vi "Dashboard Main.vi"() -> ()   [LabVIEW 2018]
uses:
  Subsystems/Drive/MotionProfile/StartingPosition.ctl
  Subsystems/Drive/MotionProfile/Path_Decider.ctl
  <vilib>/Utility/miscctls.llb/LVRowAndColumnTypeDef.ctl
  <vilib>/event_ctls.llb/eventvkey.ctl
  <vilib>/Rock Robotics/Network Tables/NT Read Numeric Array.vi
  <vilib>/Rock Robotics/Network Tables/NT Read Boolean.vi
  <vilib>/Rock Robotics/Network Tables/NT Write Variant.vi
  <vilib>/Rock Robotics/WPI/Dashboard/WPI_DashboardLogging Global.vi
panel:
  out "lineIRRearRight":bool
  out "lineIRRearLeft":bool
  out "lineIRFrontRight":bool
  out "lineIRFrontLeft":bool
  out "climbSkidIRRight":bool
  out "climbSkidIRLeft":bool
  out "climbPoweredIRLeft":bool
  out "climbPoweredIRRight":bool
  in  "Camera Settings Right":T1={"Frame Rate"=30, "Compression"=30, "Size"=1, "DB Camera Config"=FALSE} {"Frame Rate" scale=1.0..30.0; "Compression" scale=100.0..-1.0; "Size" items=["640x480", "320x240", "160x120"]}
  in  "Camera Name Right":string(combo)="No Camera Selection"
  out "Camera Perf":string
  in  "Camera Settings":T1={"Frame Rate"=30, "Compression"=30, "Size"=1, "DB Camera Config"=FALSE} {"Frame Rate" scale=1.0..30.0; "Compression" scale=100.0..-1.0; "Size" items=["640x480", "320x240", "160x120"]}
  in  "TCP":refnum<k5>
  in  "Rec Mode":enum32{"Stop", "Record", "Playback"}(radio)
  out "Robot IP":string
  out "Image Message":string="Timeout in Camera Communications"
  in  "Dashboard Tab":T2(tab)
  in  "Select Auto":string(combo)="Select Autonomous ..."
  out "NT Connection":bool
  out "MotorChart R":cluster{"Numeric":dbl, "Numeric":dbl}(graph)
  out "MotorChart L":cluster{"Numeric":dbl, "Numeric":dbl}(graph)
  out "MotorSliders R":cluster{"MotorSlide1":dbl, "MotorSlide2":dbl} {"MotorSlide2" scale=-1.0..1.0 scale format="%#_2e"; "MotorSlide1" scale=-1.0..1.0 scale format="%#_2e"}
  out "MotorSliders L":cluster{"MotorSlide1":dbl, "MotorSlide2":dbl} {"MotorSlide2" scale=-1.0..1.0 scale format="%#_2e"; "MotorSlide1" scale=-1.0..1.0 scale format="%#_2e"}
  out "Gyro":dbl(knob) scale=0.0..360.0
  out "JS1 Z":dbl(slide) scale=-1.0..1.0 scale format="%#_2e"
  out "JS1 Graph":cluster{"X":dbl, "Y":dbl}[](graph)
  out "JS1 Buttons":T3
  out "JS2 Z":dbl(slide) scale=-1.0..1.0 scale format="%#_2e"
  out "JS2 Graph":cluster{"X":dbl, "Y":dbl}[](graph)
  out "JS2 Buttons":T3
  out "Mode":T4(ring)=enum."Auto Disabled"
  out "Right Camera Perf":cluster{"Bandwidth (Mbps)":dbl, "FPS":dbl}
  out "Camera Image Right":T5(plugin-control)
  in  "DB/String 9":string
  in  "DB/String 8":string
  in  "DB/String 7":string
  in  "DB/String 6":string
  in  "DB/String 5":string
  in  "DB/String 4":string
  in  "DB/String 3":string
  in  "DB/String 2":string
  in  "DB/String 1":string
  in  "DB/String 0":string
  in  "DB/Slider 0":dbl(slide) scale=0.0..5.0
  in  "DB/Slider 1":dbl(slide) scale=0.0..5.0
  in  "DB/Slider 2":dbl(slide) scale=0.0..5.0
  in  "DB/Slider 3":dbl(slide) scale=0.0..5.0
  out "DB/LED 3":bool
  out "DB/LED 2":bool
  out "DB/LED 1":bool
  out "DB/LED 0":bool
  in  "DB/Button 3":bool
  in  "DB/Button 2":bool
  in  "DB/Button 1":bool
  in  "DB/Button 0":bool caption="New Name"
  in  "Auto Options":T8={"Starting Position"=enum."Left L1 ", "First Score Pos"=enum."7", "Second Score Pos"=enum."5"}
  out "Waveform Chart":dbl(graph)
  out "HatchPanelDetect":bool
  in  "Test Slider":dbl(slide) scale=0.0..100.0 scale format="%#_3g"
  in  "On/Off":bool caption="Solenoid"
  in  "Test Name":u16(ring) items=["Select the test to run..."]
  in  "Test Tree":string(tree)
  in  "Motor":cluster{"Value":dbl, "Enable":bool} {"Value" scale=-1.0..1.0 scale format="%#_3g"}
  out "Progress":T9 {"Test Progress" scale=0.0..100.0}
  in  "Rev/Fwd":cluster{"Forward":bool, "Reverse":bool}
  in  "Test Ring":u16(ring) items=["Monochrome", "Color"]
  out "Cmd Status":string
  in  "Execute Command":bool
  in  "Command Params":string[][](table)
  in  "Command Selection":i32(listbox)
  in  "CheckList":i32(listbox)
  out "Tree":string(tree)
  out "Camera Image":T5(plugin-control)
  out "Background":bool
  in  "Camera Name":string(combo)="No Camera Selection"
  # "HW"
  # "HW"
  # "Joysticks"
  # "Drive Motors"
  # "Front"
  # "Right"
  # "Left"
  # "Back"
  # "This tab is a great place for autonomous settings and robot-specific values.\nPlace controls and indicators inside this tab and match name to\nDashboard Variables on robot. You can also delete this comment."
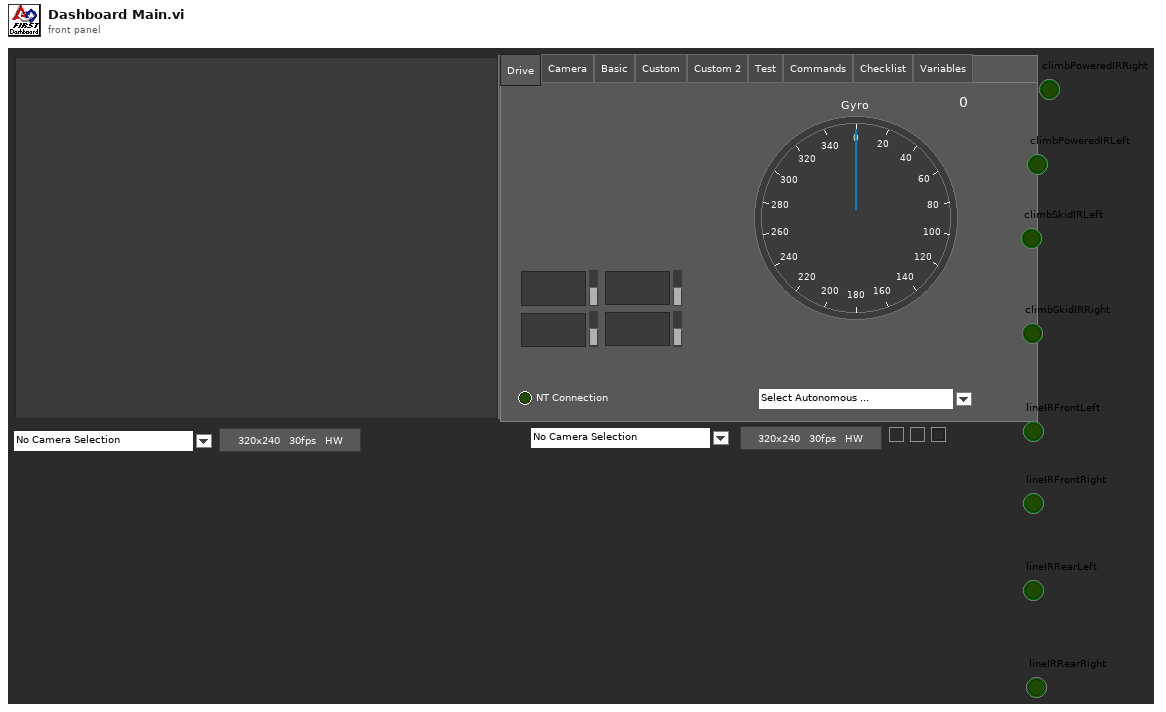
[diagram p1: front panel]
types:
  T1 = cluster{"Frame Rate":i32, "Compression":i32, "Size":u16, "DB Camera Config":bool}
  T2 = enum32{"Drive", "Camera", "Basic", "Custom", "Custom 2", "Test", "Commands", "Checklist", "Variables"}
  T3 = cluster{bool, bool, bool, bool, bool, bool, bool, bool, bool, bool, bool, bool}
  T4 = enum8{"Tele-Op Disabled", "Tele-Op Enabled", "Auto Disabled", "Auto Enabled", "Test Disabled", "Test Enabled", "Disconnected", "No Code", "E-Stop"}
  T5 = typedef "IMAQ Image.ctl" = refnum<image>
  T6 = typedef "StartingPosition.ctl" = enum16{"Left L1 ", "Middle L1", "Right L1", "Left L2", "Right L2", "Don't Move"}
  T7 = typedef "Path_Decider.ctl" = enum16{"1", "2", "3", "4", "5", "6", "7", "8", "Left_Rocket_Front", "Left_Rocket_Rear", "Right_Rocket_Front", "Right_Rocket_Rear"}
  T8 = cluster{"Starting Position":T6, "First Score Pos":T7, "Second Score Pos":T7}
  T9 = cluster{"Test Progress":u8, "Test Progress Text":string}
  T10 = cluster{"Save Path":path, "Interval (s)":dbl, "Keep":i32}
  T11 = enum32{"Drive", "Camera", "Basic", "Custom", "Test", "Commands", "Checklist", "Variables"}
  T12 = typedef "Image Type" = u32
  T13 = cluster{"IDs":cluster{"RPC field ID":u16, "Unique ID":u16}, "String":string}
  T14 = cluster{"Error Strings":string, "Disable Counts":cluster{u16, u16}, "Rail Faults":cluster{u16, u16, u16}, "Robot IP":string, "DB Mode":u8, "Event Info":cluster{"Name":string, "Type":u8, "Number":u16, "Replay":u8}}
  T15 = cluster{"Storage":cluster{"Disk Free":u64, "RAM Block":u32, "RAM free":u32}, "CPU Utilization":cluster{"CPU % ISR":sgl, "CPU % Time Crit":sgl, "CPU % Timed Str":sgl, "CPU % High":sgl, "CPU % Above":sgl, "CPU % Normal":sgl, "CPU % Low":sgl}, "CAN":cluster{"% Bus Utilization":sgl, "Bus Off Cnt":u32, "TX_FIFO Full Cnt":u32, "Receive Error Cnt":u8, "Transmit Error Cnt":u8}, "HID":cluster{"HID Outputs":u32, "Rumble Low":u16, "Rumble High":u16}[]}
  T16 = cluster{"Status bits":cluster{"Test Mode":bool, "Autonomous":bool, "Enabled":bool, "Code Start":bool, "Brownout":bool, "Reserved 2":bool, "Reserved 3":bool, "E-Stop":bool}, "Code Trace":cluster{"Disabled":bool, "TeleOp":bool, "Auto":bool, "Test":bool}, "Controller Type":enum16{"unknown", "cRIO", "roboRio"}, "Code?":enum16{"unknown", "noCode", "code"}, "Battery V":dbl}
  T17 = cluster{"Control Bits":cluster{"TestMode":bool, "Autonomous":bool, "Enabled":bool, "FMS Present":bool, bool, bool, bool, "E-Stop":bool}, "Team Station ":u8, "Countdown":sgl, "Joystick Values":cluster{"Axes":dbl[], "Buttons":bool[], "POVs":i16[]}[]}
  T18 = cluster{"Axes":dbl[], "Buttons":bool[], "POVs":i16[]}[]
  T19 = cluster{"Axes":dbl[], "Buttons":bool[], "POVs":i16[]}
  T20 = cluster{"Buttons[0]":bool, "Buttons[1]":bool, "Buttons[2]":bool, "Buttons[3]":bool, "Buttons[4]":bool, "Buttons[5]":bool, "Buttons[6]":bool, "Buttons[7]":bool, "Buttons[8]":bool, "Buttons[9]":bool, "Buttons[10]":bool, "Buttons[11]":bool}
  T21 = cluster{"Camera Image":refnum<vi>, "Dashboard Tab":refnum<vi>, "Background":refnum<vi>, "Rec Mode":refnum<vi>, "Test Slider":refnum<vi>, "On/Off ":refnum<vi>, "Test Ring":refnum<vi>, "Rev/Fwd":refnum<vi>, "Test Name":refnum<vi>, "Motor":refnum<vi>, "Progress":refnum<vi>, "CheckList":refnum<vi>, "Tree":refnum<vi>, "Test Tree":refnum<vi>, "Command Params":refnum<vi>, "Command Selection":refnum<vi>, "Execute Command":refnum<vi>, "Cmd Status":refnum<vi>, "Camera Settings":refnum<vi>, "Camera Name":refnum<vi>, "Camera Perf":refnum<vi>, "Camera Settings Right":refnum<vi>, "Camera Name Right":refnum<vi>, "Camera Image Right":refnum<vi>}
  T22 = cluster{"Global Rectangle":i32[], "Contours":cluster{"Contour Type":u32, "ROI Type":u32, "Points":i32[]}[]}
  T23 = cluster{"Camera Name Right":string, string, "Saved DB Images Info":cluster{"Save Path":path, "Interval (s)":dbl, "Keep":i32}}
  T24 = cluster{"Camera Name":string, string, "Saved DB Images Info":cluster{"Save Path":path, "Interval (s)":dbl, "Keep":i32}}
  T25 = cluster{"Operation":enum16{"Update", "Clear"}, "Color Box":u32}[]
  T26 = typedef "eventvkey.ctl" = enum16{"ASCII", "Enter", "Return", "Shift", "Ctrl", "Alt", "Cmd", "Opt", "Caps", "NumLock", "Clear", "Break", "Up", "Down", "Left", "Right", "Insert", "Delete", "Home", "End", "PageUp", "PageDown", "Escape", "Help", "Pause", "ScrollLock", "F1", "F2", "F3", "F4", "F5", "F6", "F7", "F8", "F9", "F10", "F11", "F12", "F13", "F14", "F15", "F16", "F17", "F18", "F19", "F20", "F21", "F22", "F23", "F24", "Play", "VolumeUp", "VolumeDown", "Mute", "Two Byte Char"}
  T27 = cluster{"Image Size":bool, "Image Type":bool, "Pixel Value":bool, "ROI Information":bool, "Zoom Factor":bool}
  T28 = cluster{"Operation":enum16{"Update", "Clear"}, "Color Box":u32}
  T29 = typedef "LVRowAndColumnTypeDef.ctl" = cluster{"Row":i32, "Column":i32}
  T30 = cluster{"Shift":bool, "Ctrl":bool, "Alt":bool, "Cmd":bool, "Opt":bool}
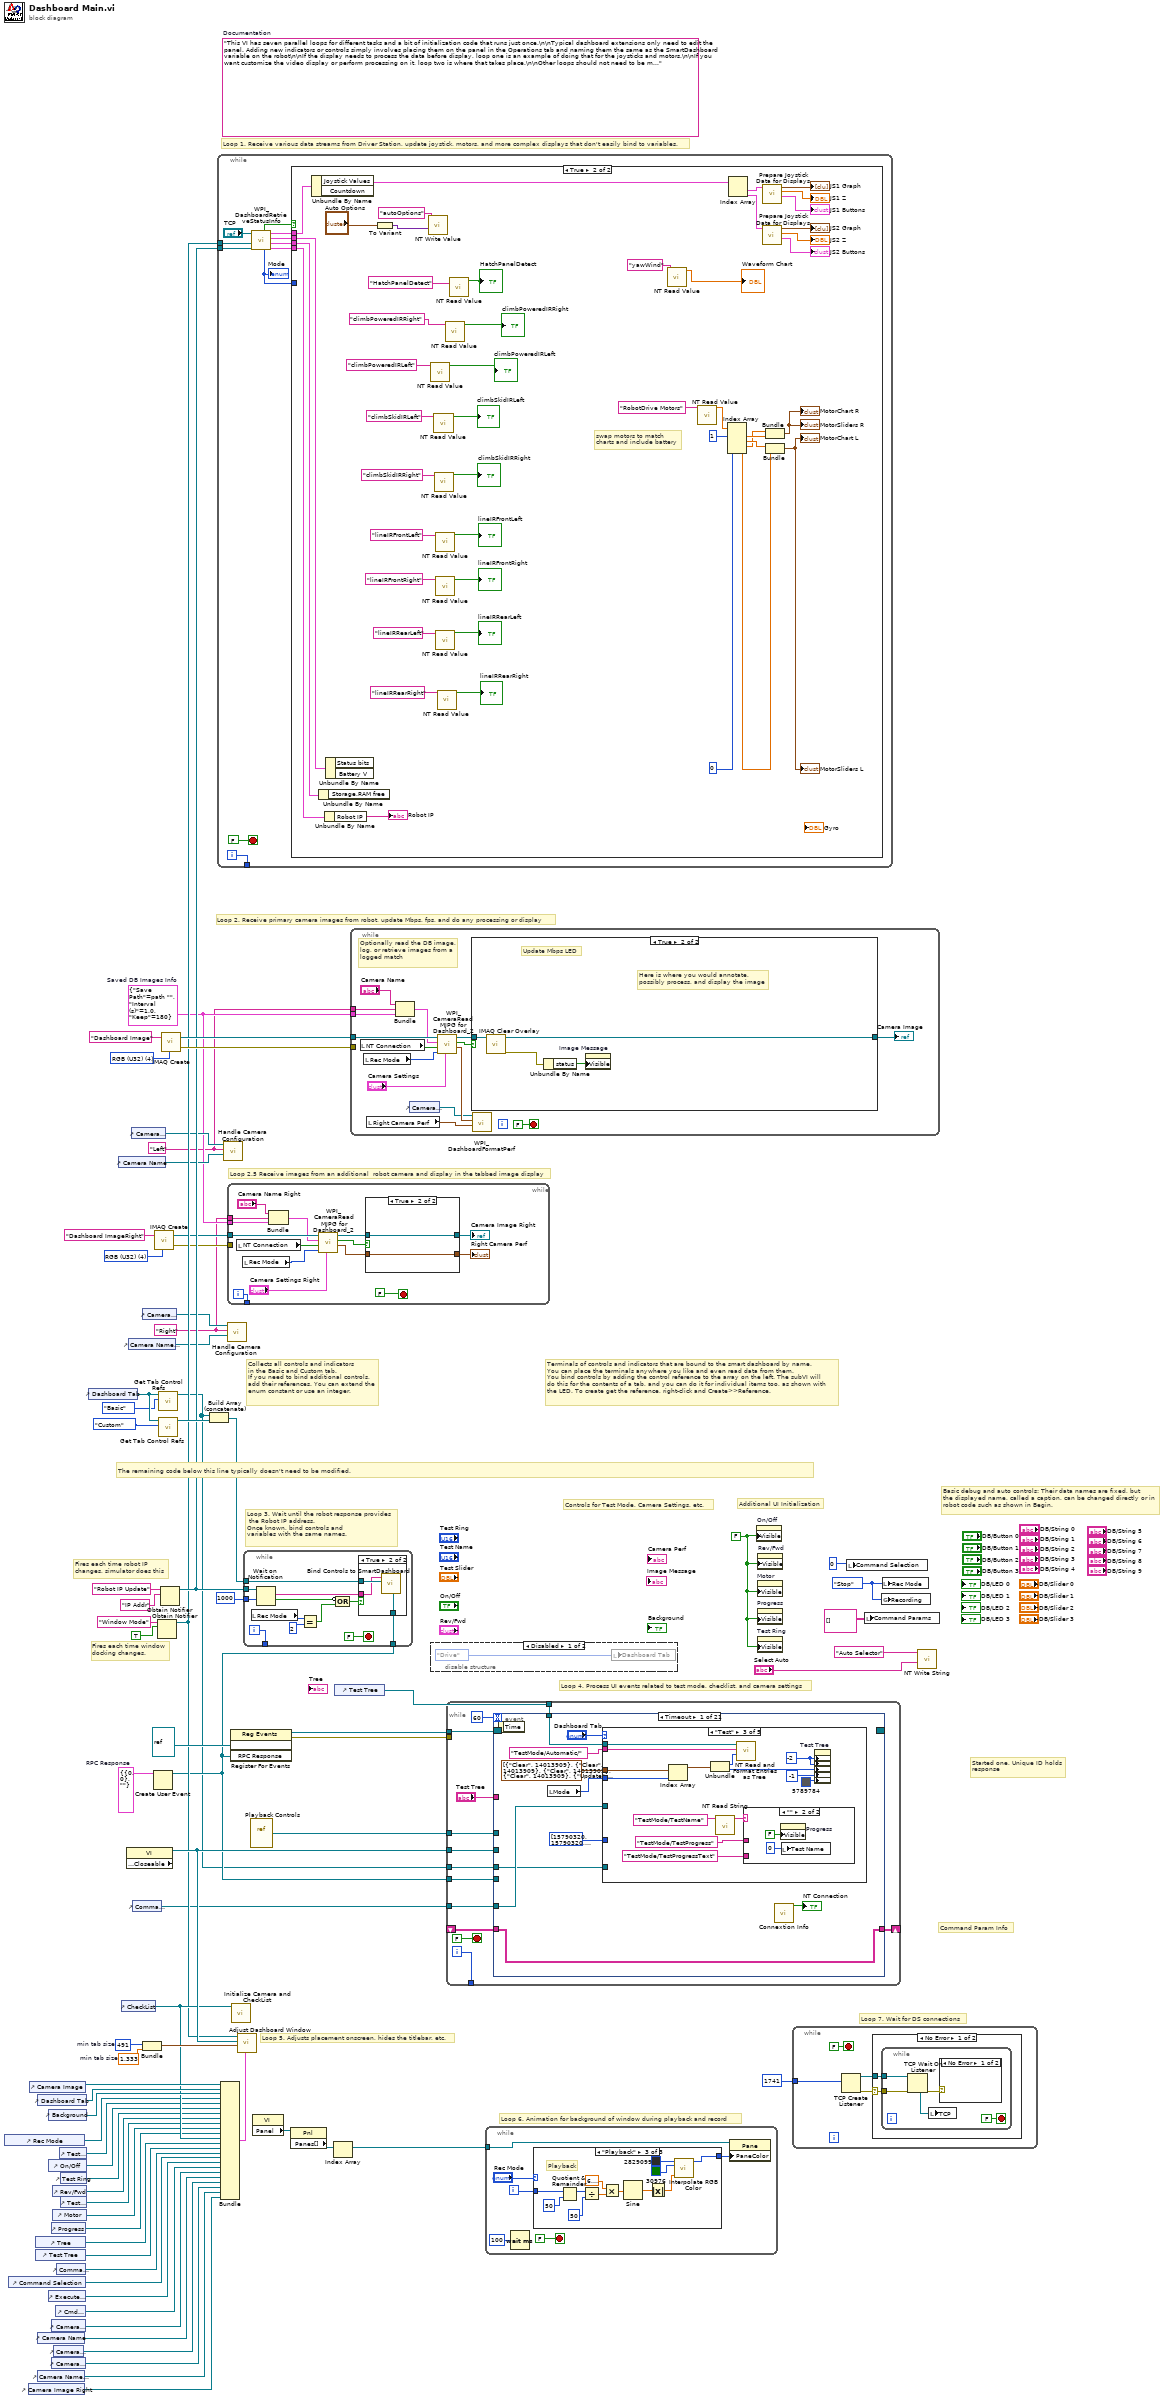
[diagram p0: block diagram]
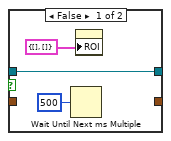
[diagram p3: hidden frame]
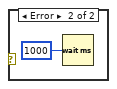
[diagram p4: hidden frame]
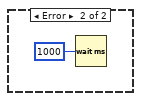
[diagram p5: hidden frame]
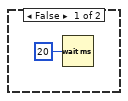
[diagram p6: hidden frame]
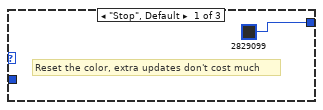
[diagram p7: hidden frame]
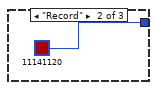
[diagram p8: hidden frame]
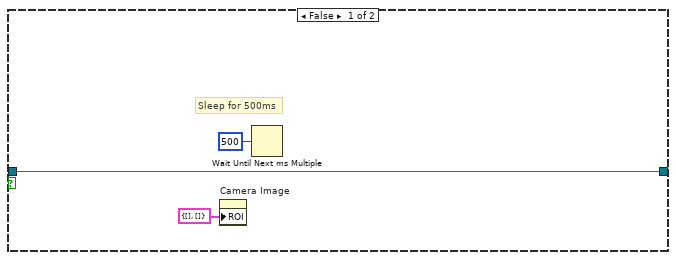
[diagram p10: hidden frame]
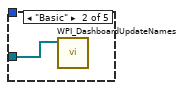
[diagram p12: hidden frame]
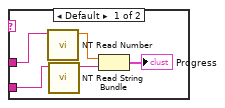
[diagram p13: hidden frame]
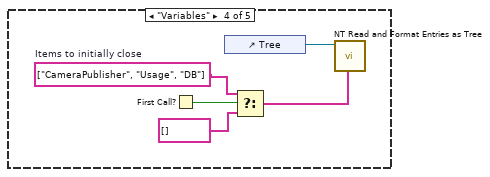
[diagram p14: hidden frame]
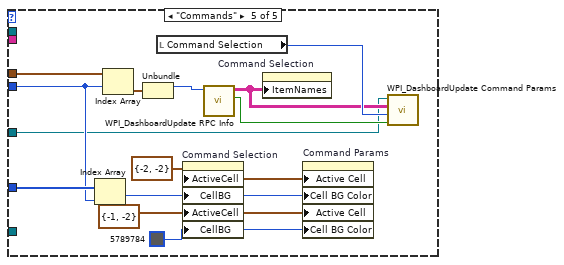
[diagram p15: hidden frame]
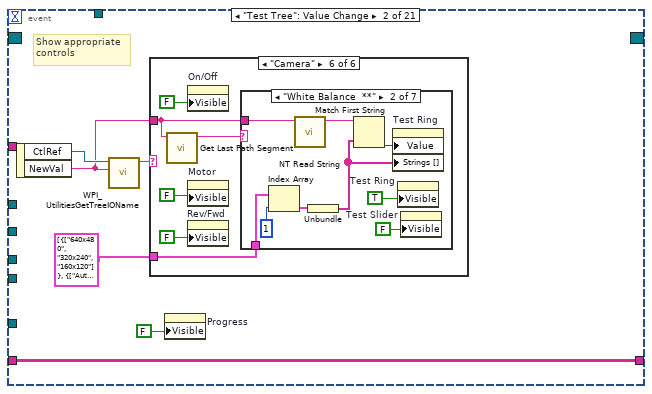
[diagram p16: hidden frame]
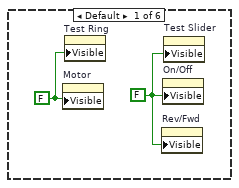
[diagram p17: hidden frame]
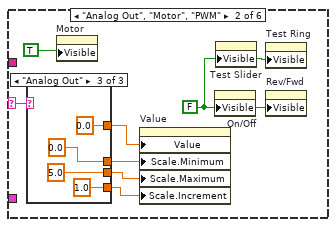
[diagram p18: hidden frame]
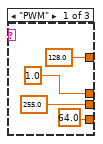
[diagram p19: hidden frame]
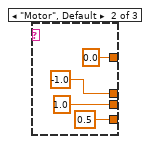
[diagram p20: hidden frame]
diagram:
  w3 = T10 {"Save Path"=path "", "Interval (s)"=1.0, "Keep"=180}  # Saved DB Images Info
  w2 = "Right"
  w1 = "Left"
  w13 = T12 4 items=["Grayscale (U8)", "Grayscale (I16)", "Grayscale (SGL)", "Complex (CSG)", "RGB (U32)", "HSL (U32)", "RGB (U64)"] ("Image Type")
  w29 = T13 {"IDs"={"RPC field ID"=0, "Unique ID"=0}, "String"=""}  # RPC Response
  w51 = 491  # min tab size
  w50 = 1.333  # min tab size
  w58 = enum32{"Stop", "Record", "Playback"}."Stop" ("Rec Mode")
  w35 = FALSE ("Visible")
  (unwired) "This VI has seven parallel loops for different tasks and a bit of initialization code that runs just once.\n\nTypical dashboard extensions only need to edit the panel. Adding new indicators or controls simply involves placing them on the panel in the Operations tab and naming them the same as the SmartDashboard variable on the robot\n\nIf the display needs to process the data before display, loop one is an example of doing that for the joysticks and motors.\n\nIf you want customize the video display or perform processing on it, loop two is where that takes place.\n\nOther loops should not need to be modified. They are pretty standard, and document the task they perform."  # Documentation
  w75 = T12 4 items=["Grayscale (U8)", "Grayscale (I16)", "Grayscale (SGL)", "Complex (CSG)", "RGB (U32)", "HSL (U32)", "RGB (U64)"] ("Image Type")
  # "Loop 2.5 Receive images from an additional  robot camera and display in the tabbed image display"
  # "Command Param Info"
  # "Started one, Unique ID holds\nresponse"
  # "Loop 7. Wait for DS connections"
  # "Basic debug and auto controls: Their data names are fixed, but\nthe displayed name, called a caption, can be changed directly or in\nrobot code such as shown in Begin."
  # "Controls for Test Mode, Camera Settings, etc."
  # "Additional UI Initialization"
  # "Loop 6. Animation for background of window during playback and record"
  # "Fires each time robot IP\nchanges, simulator does this"
  # "Fires each time window\ndocking changes."
  # "Collects all controls and indicators\nin the Basic and Custom tab.\nIf you need to bind additional controls,\nadd their references. You can extend the\nenum constant or use an integer."
  # "The remaining code below this line typically doesn't need to be modified."
  # "Loop 4. Process UI events related to test mode, checklist, and camera settings"
  # "Terminals of controls and indicators that are bound to the smart dashboard by name.\nYou can place the terminals anywhere you like and even read data from them.\nYou bind controls by adding the control reference to the array on the left. The subVI will\ndo this for the contents of a tab, and you can do it for individual items too, as shown with\nthe LED. To create get the reference, right-click and Create>>Reference."
  # "Loop 3. Wait until the robot response provides\n the Robot IP address.\nOnce known, bind controls and\nvariables with the same names."
  # "Loop 5. Adjusts placement onscreen, hides the titlebar, etc."
  # "Loop 1. Receive various data streams from Driver Station, update joystick, motors, and more complex displays that don't easily bind to variables."
  # "Loop 2. Receive primary camera images from robot, update Mbps, fps, and do any processing or display"
  n1 = control-ref of="Rec Mode"() -> (w41:refnum<vi>)
  n2 = control-ref of="Command Selection"() -> (w28:refnum<vi>)
  n3 = control-ref of="Camera Image Right"() -> (w6:refnum<vi>)
  n4 = control-ref of="Camera Image"() -> (w53:refnum<vi>)
  n5 = control-ref of="Tree"() -> (w45:refnum<vi>)
  n6 = control-ref of="Test Tree"() -> (w44:refnum<vi>)
  n7 = control-ref of="Dashboard Tab"() -> (w52:refnum<vi>)
  n8 = control-ref of="Camera Name"() -> (w19:refnum<vi>)
  n9 = control-ref of="Camera Name Right"() -> (w7:refnum<vi>)
  n10 = control-ref of="Execute Command"() -> (w30:refnum<vi>)
  n11 = control-ref of="Background"() -> (w48:refnum<vi>)
  n12 = control-ref of="On/Off"() -> (w39:refnum<vi>)
  n13 = control-ref of="Progress"() -> (w36:refnum<vi>)
  n14 = control-ref of="Camera Settings"() -> (w20:refnum<vi>)
  n15 = control-ref of="Camera Settings Right"() -> (w8:refnum<vi>)
  n16 = control-ref of="Rev/Fwd"() -> (w37:refnum<vi>)
  n17 = control-ref of="Motor"() -> (w42:refnum<vi>)
  n18 = control-ref of="Camera Perf"() -> (w18:refnum<vi>)
  n19 = control-ref of="Cmd Status"() -> (w24:refnum<vi>)
  n20 = control-ref of="Command Params"() -> (w31:refnum<vi>)
  n21 = control-ref of="Test Slider"() -> (w40:refnum<vi>)
  n22 = control-ref of="Test Ring"() -> (w38:refnum<vi>)
  n23 = control-ref of="Test Name"() -> (w43:refnum<vi>)
  n24 = control-ref of="Dashboard Tab"() -> (w56:refnum<vi>)
  n25 = control-ref of="Camera Name"() -> (w21:refnum<vi>)
  n26 = control-ref of="CheckList"() -> (w46:refnum<vi>)
  n27 = property class="VI" props=["Front Panel.Closeable"]() -> (reference out=w57:refnum<vi>)  [unwired: 2 in, 2 out]
  n28 = control-ref of="Camera Name Right"() -> (w9:refnum<vi>)
  n29 = control-ref of="Camera Settings"() -> (w22:refnum<vi>)
  n30 = control-ref of="Command Params"() -> (w23:refnum<vi>)
  n31 = control-ref of="Camera Settings Right"() -> (w10:refnum<vi>)
  n32 = Bundle("min tab size"=w51, "min tab size"=w50) -> (w49:cluster{"min tab size":i32, "min tab size":dbl})  [unwired: 1 in]
  n33 = Create User Event(user event datatype=w29) -> (user event=w25:refnum<user-event>)  [unwired: 1 in, 1 out]
  n34 = call "IMAQ Create"("Image Name"="Dashboard ImageRight", "Image Type"=w13) -> ("New Image"=w12:T5, "error out"=w11:errorcluster)  [unwired: 2 in, 1 out]
  n35 = Obtain Notifier(name (unnamed)="Window Mode", notification data type=TRUE) -> (notifier out=w33:refnum<notifier>)  [unwired: 2 in, 2 out]
  n36 = call <vilib>:"Get Tab Control Refs.vi"("Page Index"=T11."Basic" ("Dashboard Tab"), "TabControl in"=w56) -> ("ControlsOnPage"=w17:refnum<vi>[])  [unwired: 9 in]
  n37 = call <vilib>:"Get Tab Control Refs.vi"("Page Index"=T11."Custom" ("Dashboard Tab"), "TabControl in"=w56) -> ("ControlsOnPage"=w55:refnum<vi>[])  [unwired: 9 in]
  n38 = Obtain Notifier(name (unnamed)="Robot IP Update", notification data type="IP Addr" ("name (unnamed)")) -> (notifier out=w34:refnum<notifier>)  [unwired: 2 in, 2 out]
  n39 = call "IMAQ Create"("Image Name"="Dashboard Image", "Image Type"=w75) -> ("New Image"=w73:T5, "error out"=w72:errorcluster)  [unwired: 2 in, 1 out]
  n40 = Build Array (concatenate)(w17, w55) -> (w54:refnum<vi>[])
  n41 = while {
    tunnel: [w85] -> _
    tunnel: w34 -> [w79]
    tunnel: w33 -> [w76]
    i -> [w85]
    stop <- FALSE stop-if-true
    n42 = call <vilib>:"WPI_DashboardRetrieveStatusInfo.vi"("Binding Refnum"=w79, "Window Mode Notifier"=w76, "TCP Cnx"="TCP") -> ("Power and Errors"=w80:T14, "Robot Metrics"=w83:T15, "Status Info"=w84:T16, "Control Info"=w81:T17, "Robot Mode"=w78:T4, "Process?"=w82:bool)  [unwired: 3 in]
    "Mode" <- w78
    n43 = case shown="True" w82 {
      tunnel: w84 -> [_ w134]
      tunnel: w83 -> [_ w133]
      tunnel: w81 -> [_ w132]
      tunnel: w80 -> [_ w131]
      tunnel: w78 -> [_ _]
      frame False {
        n44 = Wait (ms)(milliseconds to wait=u32 20) -> ()  [unwired: 1 out]
      }
      frame True {
        # "swap motors to match\ncharts and include battery"
        n45 = Unbundle By Name(w132) -> ("Joystick Values"=w122:T18)  [unwired: 1 out]
        n46 = Unbundle By Name(w133) -> ()  [unwired: 1 out]
        n47 = Unbundle By Name(w131) -> ("Robot IP"=→"Robot IP":string)
        n48 = Unbundle By Name(w134) -> ()  [unwired: 2 out]
        n49 = To Variant(anything="Auto Options") -> (Variant=w88:variant)
        n50 = call-poly <vilib>:"NT Write Value.vi"("Variant"=w88, "Name"="autoOptions") -> ()  [unwired: 9 in, 1 out]
        n51 = call-poly <vilib>:"NT Read Value.vi"("Name"="climbPoweredIRLeft") -> ("Boolean"=→"climbPoweredIRLeft":bool)  [unwired: 9 in, 1 out]
        n52 = call-poly <vilib>:"NT Read Value.vi"("Name"="climbSkidIRLeft") -> ("Boolean"=→"climbSkidIRLeft":bool)  [unwired: 9 in, 1 out]
        n53 = call-poly <vilib>:"NT Read Value.vi"("Name"="climbSkidIRRight") -> ("Boolean"=→"climbSkidIRRight":bool)  [unwired: 9 in, 1 out]
        n54 = call-poly <vilib>:"NT Read Value.vi"("Name"="lineIRFrontLeft") -> ("Boolean"=→"lineIRFrontLeft":bool)  [unwired: 9 in, 1 out]
        n55 = call-poly <vilib>:"NT Read Value.vi"("Name"="lineIRFrontRight") -> ("Boolean"=→"lineIRFrontRight":bool)  [unwired: 9 in, 1 out]
        n56 = call-poly <vilib>:"NT Read Value.vi"("Name"="lineIRRearLeft") -> ("Boolean"=→"lineIRRearLeft":bool)  [unwired: 9 in, 1 out]
        n57 = call-poly <vilib>:"NT Read Value.vi"("Name"="lineIRRearRight") -> ("Boolean"=→"lineIRRearRight":bool)  [unwired: 9 in, 1 out]
        n58 = call-poly <vilib>:"NT Read Value.vi"("Name"="climbPoweredIRRight") -> ("Boolean"=→"climbPoweredIRRight":bool)  [unwired: 9 in, 1 out]
        n59 = call-poly <vilib>:"NT Read Value.vi"("Name"="HatchPanelDetect") -> ("Boolean"=→"HatchPanelDetect":bool)  [unwired: 9 in, 1 out]
        n60 = call-poly <vilib>:"NT Read Value.vi"("Name"="yawWind") -> ("Numeric"=→"Waveform Chart":dbl)  [unwired: 9 in, 1 out]
        n61 = call-poly <vilib>:"NT Read Value.vi"("Name"="RobotDrive Motors") -> ("Numeric Array"=w112:dbl[])  [unwired: 9 in, 1 out]
        n62 = Index Array(array=w112, index #1=1, index #4=0) -> (element #1=w126:dbl, element #2=w127:dbl, element #3=w125:dbl, element #4=w130:dbl)  [unwired: 2 in]
        n63 = Index Array(array=w122) -> (element #1=w121:T19, element #2=w117:T19)  [unwired: 2 in]
        n64 = call "Prepare Joystick Data for Displays.vi"("Joystick Values"=w117) -> ("Buttons"=→"JS2 Buttons":T20, "Z Axis"=→"JS2 Z":dbl, "Cartesian Data"=→"JS2 Graph":cluster{"X axis":dbl, "X axis":dbl}[])  [unwired: 8 in]
        n65 = call "Prepare Joystick Data for Displays.vi"("Joystick Values"=w121) -> ("Buttons"=→"JS1 Buttons":T20, "Z Axis"=→"JS1 Z":dbl, "Cartesian Data"=→"JS1 Graph":cluster{"X axis":dbl, "X axis":dbl}[])  [unwired: 8 in]
        n66 = Bundle("Numeric"=w125, "Numeric"=w126) -> (→"MotorChart R" →"MotorSliders R":cluster{"Numeric":dbl, "Numeric":dbl})  [unwired: 1 in]
        n67 = Bundle("Numeric"=w127, "Numeric"=w130) -> (→"MotorChart L" →"MotorSliders L":cluster{"Numeric":dbl, "Numeric":dbl})  [unwired: 1 in]
      }
    }
  }
  n68 = Bundle("Camera Image"=w53, "Dashboard Tab"=w52, "Background"=w48, "Rec Mode"=w41, "Test Slider"=w40, "On/Off"=w39, "Test Ring"=w38, "Rev/Fwd"=w37, "Test Name"=w43, "Motor"=w42, "Progress"=w36, "CheckList"=w46, "Tree"=w45, "Test Tree"=w44, "Command Params"=w31, "Command Selection"=w28, "Execute Command"=w30, "Cmd Status"=w24, "Camera Settings"=w20, "Camera Name"=w19, "Camera Perf"=w18, "Camera Settings Right"=w8, "Camera Name Right"=w7, "Camera Image Right"=w6) -> (w47:T21)  [unwired: 1 in]
  n69 = call "Handle Camera Configuration.vi"("CameraNameRef"=w21, "Display Name"=w1, "ClusterRef"=w22) -> ()  [unwired: 9 in]
  n70 = call "Handle Camera Configuration.vi"("CameraNameRef"=w9, "Display Name"=w2, "ClusterRef"=w10) -> ()  [unwired: 9 in]
  n71 = while {
    tunnel: w12 -> [w149]
    tunnel: w11 -> [_]
    tunnel: [w144] -> _
    tunnel: w3 -> [w140]
    tunnel: w2 -> [w137]
    i -> [w144]
    stop <- FALSE stop-if-true
    n72 = local read "NT Connection"() -> (w141:bool)
    n73 = local read "Rec Mode"() -> (w148:enum32{"Stop", "Record", "Playback"})
    n74 = Bundle("Camera Name Right"="Camera Name Right", w137, "Saved DB Images Info"=w140) -> (w139:T23)  [unwired: 1 in]
    n75 = call <vilib>:"WPI_CameraRead MJPG for Dashboard_2.vi"("Camera Settings"="Camera Settings Right", "Rec Mode"=w148, "NT Connection"=w141, "Capture Info"=w139, "Image in"=w149) -> ("perf info"=w135:cluster{"Bandwidth (Mbps)":dbl, "fps":dbl}, "Active"=w143:bool, "Image\\ out"=w146:T5)  [unwired: 4 in]
    n76 = case shown="True" w143 {
      tunnel: w146 -> [w151 w154]
      tunnel: [w151 w154] -> w142
      tunnel: [_ w153] -> w136
      tunnel: w135 -> [_ w153]
      frame False {
        n77 = Wait Until Next ms Multiple(millisecond multiple=u32 500) -> ()  [unwired: 1 out]
        n78 = property on="Camera Image Right" class="ImageControl"("ROI"=T22 {"Global Rectangle"=[], "Contours"=[]}) -> ()  [unwired: 2 in, 2 out]
      }
      frame True {
      }
    }
    "Camera Image Right" <- w142
    "Right Camera Perf" <- w136
  }
  n79 = register-events(refnum<vi> refnum, w25) -> (reference out=w62:refnum<event-registration>, error out=w61:errorcluster)  [unwired: 2 in]
  n80 = call "Initialize Camera and CheckList.vi"("ListBox in"=w46) -> ()  [unwired: 11 in]
  n81 = call "Adjust Dashboard Window.vi"("Sizing Refnums"=w47, "Size Constraints"=w49, "VI"=w57, "WIn Mode"=w33) -> ()  [unwired: 8 in]
  n82 = while {
    tunnel: w54 -> [w166]
    tunnel: w34 -> [w164]
    tunnel: [w162] -> _
    tunnel: u32 1000 ("milliseconds to wait") -> [w161]
    tunnel: w25 -> [w155]
    i -> [w162]
    stop <- FALSE stop-if-true
    n83 = local read "Rec Mode"() -> (w157:enum32{"Stop", "Record", "Playback"})
    n84 = Wait on Notification(notifier=w164, timeout in ms (-1)=w161) -> (notification=w163:string, timed out?=w159:bool)  [unwired: 2 in, 2 out]
    n85 = Equal?(x=w157, y=u16 2 ("Rec Mode")) -> (x = y?=w158:bool)
    n86 = Compound Arithmetic op=OR(invert w159, w158) -> (w160:bool)
    n87 = case shown="True" w160 {
      tunnel: w166 -> [_ w169]
      tunnel: w163 -> [_ w168]
      tunnel: w155 -> [_ w167]
      frame False {
      }
      frame True {
        n88 = call <vilib>:"Bind Controls to SmartDashboard.vi"("RPC ref"=w167, "Bound Control Refs"=w169, "Server IP Address"=w168) -> ()  [unwired: 9 in]
      }
    }
  }
  n89 = vi-ref "Playback Controls.vi"() -> (w63:refnum<vi>)
  n90 = property class="VI"() -> ("Panel"=w65:refnum<vi>)  [unwired: 2 in, 2 out]
  n91 = property class="Pnl"(reference=w65) -> ("Panes[]"=w66:refnum<vi>[])  [unwired: 1 in, 2 out]
  n92 = Index Array(array=w66) -> (element=w64:refnum<vi>)  [unwired: 1 in]
  n93 = control-ref of="Test Tree"() -> (w67:refnum<vi>)
  n94 = while {
    tunnel: w73 -> [w183]
    tunnel: w72 -> [_]
    tunnel: w3 -> [w176]
    tunnel: w1 -> [w173]
    stop <- FALSE stop-if-true
    # "Optionally read the DB image,\nlog, or retrieve images from a\nlogged match"
    n95 = local read "NT Connection"() -> (w177:bool)
    n96 = local read "Rec Mode"() -> (w180:enum32{"Stop", "Record", "Playback"})
    n97 = local read "Right Camera Perf"() -> (w171:cluster{"Bandwidth (Mbps)":dbl, "FPS":dbl})
    n98 = Bundle("Camera Name"="Camera Name", w173, "Saved DB Images Info"=w176) -> (w175:T24)  [unwired: 1 in]
    n99 = control-ref of="Camera Perf"() -> (w170:refnum<vi>)
    n100 = call <vilib>:"WPI_CameraRead MJPG for Dashboard_2.vi"("Camera Settings"="Camera Settings", "Rec Mode"=w180, "NT Connection"=w177, "Capture Info"=w175, "Image in"=w183) -> ("perf info"=w172:cluster{"Bandwidth (Mbps)":dbl, "fps":dbl}, "Active"=w181:bool, "Image\\ out"=w182:T5)  [unwired: 4 in]
    n101 = case shown="True" w181 {
      tunnel: w182 -> [w186 w189]
      tunnel: [w186 w188] -> w178
      frame False {
        # "Sleep for 500ms"
        n102 = property on="Camera Image" class="ImageControl"("ROI"=T22 {"Global Rectangle"=[], "Contours"=[]}) -> ()  [unwired: 2 in, 2 out]
        n103 = Wait Until Next ms Multiple(millisecond multiple=u32 500) -> ()  [unwired: 1 out]
      }
      frame True {
        # "Here is where you would annotate,\npossibly process, and display the image"
        # "Update Mbps LED"
        n104 = call "IMAQ Clear Overlay"("Image"=w189) -> ("error out"=w190:errorcluster, "Image Out"=w188:T5)  [unwired: 2 in, 7 out]
        n105 = Unbundle By Name(w190) -> ("status"=w191:bool)
        n106 = property on="Image Message" class="Str"("Visible"=w191) -> ()  [unwired: 2 in, 2 out]
      }
    }
    "Camera Image" <- w178
    n107 = call <vilib>:"WPI_DashboardFormatPerf.vi"("Right Camera Perf"=w171, "Performance"=w172, "String in"=w170) -> ()  [unwired: 9 in]
  }
  n108 = disable-structure shown="Disabled" {
    frame Disabled {
      n109 = local write "Dashboard Tab"(T11."Drive" ("Dashboard Tab")) -> ()
    }
    frame Enabled {
    }
  }
  n110 = while {
    tunnel: [w202] -> _
    tunnel: w67 -> [w201]
    tunnel: w63 -> [w200]
    tunnel: w62 -> [w199]
    tunnel: w61 -> [_]
    tunnel: w57 -> [w198]
    tunnel: w25 -> [w197]
    tunnel: w23 -> [w196]
    shift-right: [w195] -> _
    shift-left: _ -> [w194]
    tunnel: w17 -> [w193]
    i -> [w202]
    stop <- FALSE stop-if-true
    n111 = event shown="[0] Timeout" {
      selector: w199 -> [_ _ _ _ _ _ _ _ _ _ _ _ _ _ _ _ _ _ _ _ _]
      dyn-events: [_ _ _ _ _ _ _ _ _ _ _ _ _ _ _ _ w462 _ _ _ _] -> _
      timeout: u32 60 ("milliseconds to wait") -> [_ _ _ _ _ _ _ _ _ _ _ _ _ _ _ _ _ _ _ _ _]
      tunnel: w201 -> [w214 _ _ _ _ _ _ _ _ _ _ _ _ _ _ _ _ _ _ _ _]
      tunnel: "Test Tree" -> [_ _ _ _ _ _ _ _ _ _ _ w429 w437 w439 w443 w451 _ _ _ _ _]
      tunnel: w200 -> [_ _ _ _ _ _ _ _ _ _ _ _ _ _ _ _ w464 _ w482 _ _]
      tunnel: w198 -> [_ _ _ _ _ _ _ _ _ _ _ _ _ _ _ _ w460 _ _ _ _]
      tunnel: w197 -> [_ _ _ _ _ _ _ _ _ _ _ _ _ _ _ _ w458 _ _ _ _]
      tunnel: w196 -> [w209 _ _ _ _ _ w380 _ _ _ _ _ _ _ _ _ _ _ _ _ _]
      tunnel: [w208 w257 w359 w364 w373 w377 w378 w387 w397 w404 w416 w428 w435 w438 w442 w450 w457 w477 w479 w483 w496] -> w195
      tunnel: w194 -> [w208 w257 w359 w364 w373 w377 w378 _ _ w404 w416 w428 w435 w438 w442 w450 w457 w477 w479 w483 w496]
      tunnel: w193 -> [w206 _ _ _ _ _ _ _ _ _ _ _ _ _ _ _ _ _ _ _ _]
      event Timeout {
        n112 = event-data() -> ()  [unwired: 1 in, 1 out]
        n113 = local read "Mode"() -> (w211:T4)
        n114 = case shown="\"Test\"" "Dashboard Tab" {
          tunnel: w214 -> [_ _ w230 _ _]
          tunnel: "TestMode/Automatic/" ("Name Pattern") -> [_ _ w229 _ _]
          tunnel: T25 [{"Operation"=enum."Clear", "Color Box"=14013909}, {"Operation"=enum."Clear", "Color Box"=14013909}, {"Operation"=enum."Clear", "Color Box"=14013909}, {"Operation"=enum."Clear", "Color Box"=14013909}, {"Operation"=enum."Update", "Color Box"=14013909}, {"Operation"=enum."Update", "Color Box"=16777215}, {"Operation"=enum."Clear", "Color Box"=14013909}, {"Operation"=enum."Clear", "Color Box"=14013909}, {"Operation"=enum."Clear", "Color Box"=14013909}] -> [_ _ w222 _ w250]
          tunnel: w211 -> [_ _ w221 _ w249]
          tunnel: u32[] [15790320, 15790320, 15790320, 15790320, 16777215, 16777215, 15790320, 15790320, 15790320] -> [_ _ _ _ w255]
          tunnel: w209 -> [_ _ _ _ w243]
          tunnel: w206 -> [_ w216 _ _ _]
          frame "Custom", Default {
          }
          frame "Basic" {
            n115 = call <vilib>:"WPI_DashboardUpdateNames.vi"("Controls on Tab"=w216) -> ()  [unwired: 11 in]
          }
          frame "Test" {
            w228 = -2 ("Active Item:Row Number")
            n116 = Index Array(array=w222, index=w221) -> (element=w223:T28)
            n117 = Unbundle(w223) -> ("Operation"=w224:enum16{"Update", "Clear"}, "Color Box"=w225:u32)
            n118 = call <vilib>:"NT Read String.vi"("Name"="TestMode/TestName") -> ("String"=w219:string)  [unwired: 9 in, 1 out]
            n119 = call <vilib>:"NT Read and Format Entries as Tree.vi"("Operation"=w224, "Name Pattern"=w229, "Tree Refnum"=w230) -> ()  [unwired: 7 in, 2 out]
            n120 = case shown="\"\"" w219 {
              tunnel: "TestMode/TestProgress" ("Name") -> [w232 _]
              tunnel: "TestMode/TestProgressText" ("Name") -> [w231 _]
              frame Default {
                n121 = call <vilib>:"NT Read Number.vi"("Name"=w232) -> ("Numeric"=w233:dbl)  [unwired: 9 in, 1 out]
                n122 = call <vilib>:"NT Read String.vi"("Name"=w231) -> ("String"=w234:string)  [unwired: 9 in, 1 out]
                n123 = Bundle("Numeric"=w233, "String"=w234) -> (→"Progress":cluster{"Numeric":dbl, "String":string})  [unwired: 1 in]
              }
              frame "" {
                n124 = property on="Progress" class="Clust (strict)"("Visible"=FALSE) -> ()  [unwired: 2 in, 2 out]
                n125 = local write "Test Name"(u16 0) -> ()
              }
            }
            n126 = property on="Test Tree" class="Tree (strict)"("Active Item Row Number"=w228, "ActiveColNum"=w228, "CellBG"=w225, "Active Item Row Number"=-1 ("Active Item:Row Number"), "CellBG"=u32 5789784 ("Color Box")) -> ()  [unwired: 2 in, 2 out]
          }
          frame "Variables" {
            w240 = string[] ["CameraPublisher", "Usage", "DB"]  # Items to initially close
            n127 = First Call?() -> (First Call?: T/F=w241:bool)
            n128 = control-ref of="Tree"() -> (w242:refnum<vi>)
            n129 = Select(t=w240, s=w241, f=string[] []) -> (s? t:f=w238:string[])
            n130 = call <vilib>:"NT Read and Format Entries as Tree.vi"("Tags to  Close"=w238, "Tree Refnum"=w242) -> ()  [unwired: 8 in, 2 out]
          }
          frame "Commands" {
            w251 = u32 5789784 ("Color Box")
            w252 = T29 {"Row"=-1, "Column"=-2} ("Active Cell:Active Cell")
            w254 = T29 {"Row"=-2, "Column"=-2} ("Active Cell:Active Cell")
            n131 = Index Array(array=w255, index=w249) -> (element=w253:u32)
            n132 = Index Array(array=w250, index=w249) -> (element=w248:T28)
            n133 = Unbundle(w248) -> ("Operation"=w247:enum16{"Update", "Clear"})  [unwired: 1 out]
            n134 = local read "Command Selection"() -> (w246:i32)
            n135 = property on="Command Selection" class="MCListbox (strict)"("ActiveCell"=w254, "CellBG"=w253, "ActiveCell"=w252, "CellBG"=w251) -> ()  [unwired: 2 in, 2 out]
            n136 = call <vilib>:"WPI_DashboardUpdate RPC Info.vi"("Operation"=w247) -> ("update"=w245:bool, "commands"=w244:string[][])  [unwired: 9 in]
            n137 = property on="Command Selection" class="MCListbox (strict)"("ItemNames"=w244) -> ()  [unwired: 2 in, 2 out]
            n138 = property on="Command Params" class="Tbl (strict)"("Active Cell"=w254, "Cell BG Color"=w253, "Active Cell"=w252, "Cell BG Color"=w251) -> ()  [unwired: 2 in, 2 out]
            n139 = call <vilib>:"WPI_DashboardUpdate Command Params.vi"("Update"=w245, "NewVal"=w246, "Commands"=w244, "Param Tbl"=w243) -> ()  [unwired: 7 in, 1 out]
          }
        }
        n140 = call <vilib>:"Connextion Info.vi"() -> ("Connected"=→"NT Connection":bool)  [unwired: 10 in, 1 out]
      }
      event "Test Tree": Value Change {
        # "Show appropriate\ncontrols"
        n141 = event-data() -> ("CtlRef"=w260:refnum<vi>, "NewVal"=w258:string)  [unwired: 1 in]
        n142 = call <vilib>:"WPI_UtilitiesGetTreeIOName.vi"("NewVal"=w258, "TreeControl in"=w260) -> ("I/O Name"=w261:string)  [unwired: 9 in]
        n143 = case shown="\"Camera\"" w261 {
          selector: w261 -> [_ w268 _ w290 w299 _]
          tunnel: w258 -> [_ _ w287 w289 _ w306]
          tunnel: cluster{string[]}[] [{["640x480", "320x240", "160x120"]}, {["Auto", "Fixed indoor", "Fixed outdoor 1", "Fixed outdoor 2", "Fixed fluorescent 1", "Fixed fluorescent 2", "Hold current"]}, {["Auto", "Flicker-free 50 Hz", "Flicker-free 60 Hz", "Hold current"]}, {["None", "Prioritize frame rate", "Prioritize image quality"]}, {["Monochrome", "Color"]}] -> [_ _ _ _ _ w305]
          frame Default {
            w263 = FALSE ("Visible")
            w262 = FALSE ("Visible")
            n144 = property on="Motor" class="Clust (strict)"("Visible"=w262) -> ()  [unwired: 2 in, 2 out]
            n145 = property on="Test Ring" class="Ring (strict)"("Visible"=w262) -> ()  [unwired: 2 in, 2 out]
            n146 = property on="Rev/Fwd" class="Clust (strict)"("Visible"=w263) -> ()  [unwired: 2 in, 2 out]
            n147 = property on="On/Off" class="Bool (strict)"("Visible"=w263) -> ()  [unwired: 2 in, 2 out]
            n148 = property on="Test Slider" class="Slide (strict)"("Visible"=w263) -> ()  [unwired: 2 in, 2 out]
          }
          frame "Analog Out", "Motor", "PWM" {
            w269 = FALSE ("Visible")
            n149 = case shown="\"Analog Out\"" w268 {
              tunnel: [1.0 ("Value") -1.0 ("Value") 0.0 ("Value")] -> w267
              tunnel: [255.0 ("Value") 1.0 ("Value") 5.0 ("Value")] -> w266
              tunnel: [128.0 ("Value") 0.0 ("Value") 0.0 ("Value")] -> w265
              tunnel: [64.0 ("Value") 0.5 ("Value") 1.0 ("Value")] -> w264
              frame "PWM" {
              }
              frame "Motor", Default {
              }
              frame "Analog Out" {
              }
            }
            n150 = property on="Motor" class="Clust (strict)"("Visible"=TRUE) -> ()  [unwired: 2 in, 2 out]
            n151 = property on="Value" class="Slide (strict)"("Value"=w265, "Scale.Minimum"=w267, "Scale.Maximum"=w266, "Scale.Increment"=w264) -> ()  [unwired: 2 in, 2 out]
            n152 = property on="On/Off" class="Bool (strict)"("Visible"=w269) -> ()  [unwired: 2 in, 2 out]
            n153 = property on="Test Slider" class="Slide (strict)"("Visible"=w269) -> ()  [unwired: 2 in, 2 out]
            n154 = property on="Test Ring" class="Ring (strict)"("Visible"=w269) -> ()  [unwired: 2 in, 2 out]
            n155 = property on="Rev/Fwd" class="Clust (strict)"("Visible"=w269) -> ()  [unwired: 2 in, 2 out]
          }
          frame "Servo" {
            w285 = FALSE ("Visible")
            n156 = call <vilib>:"NT Read Number.vi"("Name"=w287) -> ("Numeric"=w286:dbl)  [unwired: 9 in, 1 out]
            n157 = property on="Test Slider" class="Slide (strict)"("Visible"=TRUE, "Scale.Maximum"=170.0 ("Scale.Range:Maximum")) -> ()  [unwired: 2 in, 2 out]
            n158 = local write "Test Slider"(w286) -> ()
            n159 = property on="Motor" class="Clust (strict)"("Visible"=w285) -> ()  [unwired: 2 in, 2 out]
            n160 = property on="Rev/Fwd" class="Clust (strict)"("Visible"=w285) -> ()  [unwired: 2 in, 2 out]
            n161 = property on="On/Off" class="Bool (strict)"("Visible"=w285) -> ()  [unwired: 2 in, 2 out]
            n162 = property on="Test Ring" class="Ring (strict)"("Visible"=w285) -> ()  [unwired: 2 in, 2 out]
          }
          frame "Relay", "Solenoid" {
            w288 = FALSE ("Visible")
            n163 = property on="Motor" class="Clust (strict)"("Visible"=w288) -> ()  [unwired: 2 in, 2 out]
            n164 = property on="Test Slider" class="Slide (strict)"("Visible"=w288) -> ()  [unwired: 2 in, 2 out]
            n165 = Search and Replace String(input string=w289, search string="/Value  **", replace string="/Direction") -> (result string=w295:string)  [unwired: 5 in, 3 out]
            n166 = property on="Test Ring" class="Ring (strict)"("Visible"=w288) -> ()  [unwired: 2 in, 2 out]
            n167 = call <vilib>:"NT Read String.vi"("Name"=w295) -> ("String"=w293:string)  [unwired: 9 in, 1 out]
            n168 = Equal?(x="Both directions", y=w293) -> (x = y?=w291:bool)
            n169 = Not(x=w291) -> (.not. x?=w292:bool)
            n170 = property on="Rev/Fwd" class="Clust (strict)"("Visible"=w291) -> ()  [unwired: 2 in, 2 out]
            n171 = property on="On/Off" class="Bool (strict)"("Visible"=w292, "Caption.Text"=w290) -> ()  [unwired: 2 in, 2 out]
          }
          frame "Compressor", "Digital Out" {
            w298 = FALSE ("Visible")
            # "Get direction and finish"
            n172 = property on="Motor" class="Clust (strict)"("Visible"=w298) -> ()  [unwired: 2 in, 2 out]
            n173 = property on="Test Slider" class="Slide (strict)"("Visible"=w298) -> ()  [unwired: 2 in, 2 out]
            n174 = property on="Test Ring" class="Ring (strict)"("Visible"=w298) -> ()  [unwired: 2 in, 2 out]
            n175 = property on="On/Off" class="Bool (strict)"("Visible"=TRUE, "Caption.Text"=w299) -> ()  [unwired: 2 in, 2 out]
            n176 = property on="Rev/Fwd" class="Clust (strict)"("Visible"=FALSE) -> ()  [unwired: 2 in, 2 out]
          }
          frame "Camera" {
            n177 = call <vilib>:"Get Last Path Segment.vi"("String in"=w306) -> ("String out"=w307:string)  [unwired: 10 in]
            n178 = property on="On/Off" class="Bool (strict)"("Visible"=FALSE) -> ()  [unwired: 2 in, 2 out]
            n179 = property on="Motor" class="Clust (strict)"("Visible"=FALSE) -> ()  [unwired: 2 in, 2 out]
            n180 = property on="Rev/Fwd" class="Clust (strict)"("Visible"=FALSE) -> ()  [unwired: 2 in, 2 out]
            n181 = case shown="\"White Balance  **\"" w307 {
              tunnel: w306 -> [w313 w322 w331 w340 w349 _ w355]
              tunnel: w305 -> [w311 w319 w328 w337 w346 _ _]
              frame "Size  **" {
                n182 = Index Array(array=w311) -> (element=w310:cluster{string[]})  [unwired: 1 in]
                n183 = call <vilib>:"NT Read String.vi"("Name"=w313) -> ("String"=w312:string)  [unwired: 9 in, 1 out]
                n184 = Unbundle(w310) -> (w308:string[])
                n185 = Match First String(2:w308, 3:w312) -> (0:w309:i32)  [unwired: 1 out]
                n186 = property on="Test Ring" class="Ring (strict)"("Value"=w309, "Strings []"=w308) -> ()  [unwired: 2 in, 2 out]
                n187 = property on="Test Ring" class="Ring (strict)"("Visible"=TRUE) -> ()  [unwired: 2 in, 2 out]
                n188 = property on="Test Slider" class="Slide (strict)"("Visible"=FALSE) -> ()  [unwired: 2 in, 2 out]
              }
              frame "White Balance  **" {
                n189 = Index Array(array=w319, index=1) -> (element=w320:cluster{string[]})
                n190 = call <vilib>:"NT Read String.vi"("Name"=w322) -> ("String"=w321:string)  [unwired: 9 in, 1 out]
                n191 = Unbundle(w320) -> (w317:string[])
                n192 = Match First String(2:w317, 3:w321) -> (0:w316:i32)  [unwired: 1 out]
                n193 = property on="Test Ring" class="Ring (strict)"("Value"=w316, "Strings []"=w317) -> ()  [unwired: 2 in, 2 out]
                n194 = property on="Test Ring" class="Ring (strict)"("Visible"=TRUE) -> ()  [unwired: 2 in, 2 out]
                n195 = property on="Test Slider" class="Slide (strict)"("Visible"=FALSE) -> ()  [unwired: 2 in, 2 out]
              }
              frame "Exposure  **" {
                n196 = Index Array(array=w328, index=2) -> (element=w329:cluster{string[]})
                n197 = call <vilib>:"NT Read String.vi"("Name"=w331) -> ("String"=w330:string)  [unwired: 9 in, 1 out]
                n198 = Unbundle(w329) -> (w325:string[])
                n199 = Match First String(2:w325, 3:w330) -> (0:w326:i32)  [unwired: 1 out]
                n200 = property on="Test Ring" class="Ring (strict)"("Value"=w326, "Strings []"=w325) -> ()  [unwired: 2 in, 2 out]
                n201 = property on="Test Ring" class="Ring (strict)"("Visible"=TRUE) -> ()  [unwired: 2 in, 2 out]
                n202 = property on="Test Slider" class="Slide (strict)"("Visible"=FALSE) -> ()  [unwired: 2 in, 2 out]
              }
              frame "Exposure Priority  **" {
                n203 = Index Array(array=w337, index=3) -> (element=w338:cluster{string[]})
                n204 = call <vilib>:"NT Read String.vi"("Name"=w340) -> ("String"=w339:string)  [unwired: 9 in, 1 out]
                n205 = Unbundle(w338) -> (w334:string[])
                n206 = Match First String(2:w334, 3:w339) -> (0:w335:i32)  [unwired: 1 out]
                n207 = property on="Test Ring" class="Ring (strict)"("Value"=w335, "Strings []"=w334) -> ()  [unwired: 2 in, 2 out]
                n208 = property on="Test Ring" class="Ring (strict)"("Visible"=TRUE) -> ()  [unwired: 2 in, 2 out]
                n209 = property on="Test Slider" class="Slide (strict)"("Visible"=FALSE) -> ()  [unwired: 2 in, 2 out]
              }
              frame "Color Enable  **" {
                n210 = Index Array(array=w346, index=4) -> (element=w347:cluster{string[]})
                n211 = call <vilib>:"NT Read String.vi"("Name"=w349) -> ("String"=w348:string)  [unwired: 9 in, 1 out]
                n212 = Unbundle(w347) -> (w343:string[])
                n213 = Match First String(2:w343, 3:w348) -> (0:w344:i32)  [unwired: 1 out]
                n214 = property on="Test Ring" class="Ring (strict)"("Value"=w344, "Strings []"=w343) -> ()  [unwired: 2 in, 2 out]
                n215 = property on="Test Ring" class="Ring (strict)"("Visible"=TRUE) -> ()  [unwired: 2 in, 2 out]
                n216 = property on="Test Slider" class="Slide (strict)"("Visible"=FALSE) -> ()  [unwired: 2 in, 2 out]
              }
              frame Default {
                n217 = property on="Test Ring" class="Ring (strict)"("Visible"=FALSE) -> ()  [unwired: 2 in, 2 out]
                n218 = property on="Test Slider" class="Slide (strict)"("Visible"=FALSE) -> ()  [unwired: 2 in, 2 out]
              }
              frame "Brightness  **", "Color Level  **", "Compression  **", "FPS  **", "Sharpness  **" {
                n219 = call <vilib>:"NT Read Number.vi"("Name"=w355) -> ("Numeric"=w354:dbl)  [unwired: 9 in, 1 out]
                n220 = local write "Test Slider"(w354) -> ()
                n221 = property on="Test Slider" class="Slide (strict)"("Visible"=TRUE, "Scale.Maximum"=100.0 ("Scale.Range:Maximum")) -> ()  [unwired: 2 in, 2 out]
                n222 = property on="Test Ring" class="Ring (strict)"("Visible"=FALSE) -> ()  [unwired: 2 in, 2 out]
              }
            }
          }
        }
        n223 = property on="Progress" class="Clust (strict)"("Visible"=FALSE) -> ()  [unwired: 2 in, 2 out]
      }
      event "Test Name": Mouse Enter {
        # "Populate the ring with the list of tests"
        n224 = event-data() -> ()  [unwired: 1 in, 1 out]
        n225 = call <vilib>:"NT Read String Array.vi"("Name"="TestMode/TestList") -> ("String Array"=w363:string[])  [unwired: 9 in, 1 out]
        n226 = Build Array (concatenate)("Select the test to run...", w363) -> (w362:string[])
        n227 = property on="Test Name" class="Ring (strict)"("Strings []"=w362) -> ()  [unwired: 2 in, 2 out]
      }
      event "Test Name": Value Change {
        w365 = FALSE ("Visible")
        # "Tell the robot the test name to run"
        n228 = event-data() -> ("NewVal"=w369:u16)  [unwired: 1 in]
        n229 = property on="Test Name" class="Ring (strict)"() -> ("Strings []"=w370:string[])  [unwired: 2 in, 2 out]
        n230 = local write "Progress"(T9 {"Test Progress"=0, "Test Progress Text"=""} ("Progress")) -> ()
        n231 = Index Array(array=w370, index=w369) -> (element=w368:string)
        n232 = call <vilib>:"NT Write String.vi"("String"=w368, "Name"="TestMode/TestName") -> ()  [unwired: 9 in, 1 out]
        n233 = property on="Progress" class="Clust (strict)"("Visible"=TRUE) -> ()  [unwired: 2 in, 2 out]
        n234 = property on="Motor" class="Clust (strict)"("Visible"=w365) -> ()  [unwired: 2 in, 2 out]
        n235 = property on="Test Slider" class="Slide (strict)"("Visible"=w365) -> ()  [unwired: 2 in, 2 out]
        n236 = property on="On/Off" class="Bool (strict)"("Visible"=w365) -> ()  [unwired: 2 in, 2 out]
        n237 = property on="Rev/Fwd" class="Clust (strict)"("Visible"=w365) -> ()  [unwired: 2 in, 2 out]
        n238 = property on="Test Ring" class="Ring (strict)"("Visible"=w365) -> ()  [unwired: 2 in, 2 out]
      }
      event "Select Auto": Mouse Enter {
        # "Populate the combo box with the list of autonomous options"
        n239 = event-data() -> ()  [unwired: 1 in, 1 out]
        n240 = call <vilib>:"NT Read String Array.vi"("Name"="Auto List") -> ("String Array"=w372:string[])  [unwired: 9 in, 1 out]
        n241 = property on="Select Auto" class="CmbBox"("Strings[]"=w372) -> ()  [unwired: 2 in, 2 out]
      }
      event "Select Auto": Value Change {
        # "User modified the Auto Selection. Write to NT variable so robot knows."
        n242 = event-data() -> ("NewVal"=w375:string)  [unwired: 1 in]
        n243 = call <vilib>:"NT Write String.vi"("String"=w375, "Name"="Auto Selector") -> ()  [unwired: 9 in, 1 out]
      }
      event "Command Selection": Value Change {
        # "Get the params and show in table"
        n244 = event-data() -> ("NewVal"=w381:i32)  [unwired: 1 in]
        n245 = property on="Command Selection" class="MCListbox (strict)"() -> ("ItemNames"=w379:string[][])  [unwired: 2 in, 2 out]
        n246 = call <vilib>:"WPI_DashboardUpdate Command Params.vi"("NewVal"=w381, "Commands"=w379, "Param Tbl"=w380) -> ()  [unwired: 8 in, 1 out]
      }
      event "Execute Command": Value Change {
        # "Started one, Unique ID holds\nresponse"
        n247 = event-data() -> ()  [unwired: 1 in, 1 out]
        n248 = property on="Command Selection" class="MCListbox (strict)"() -> ("ItemNames"=w392:string[][])  [unwired: 2 in, 2 out]
        n249 = Index Array(array=w392, index (row)="Command Selection", index (col)=0) -> (element=w390:string)
        n250 = call <vilib>:"Invoke Commands.vi"("Command Params"="Command Params", "Function Name"=w390) -> ("Params"=w386:u8, "Started"=w385:bool)  [unwired: 7 in, 1 out]
        n251 = Array Subset(array="Command Params", length (row)=w386) -> (w387:string[][])  [unwired: 3 in]
        n252 = Select(t="Executing" ("Cmd Status"), s=w385, f="" ("Cmd Status")) -> (s? t:f=→"Cmd Status":string)
      }
      event "Command Selection": Double Click {
        n253 = event-data() -> ("Row"=w400:i32)  [unwired: 1 in]
        n254 = property on="Command Selection" class="MCListbox (strict)"() -> ("ItemNames"=w403:string[][])  [unwired: 2 in, 2 out]
        n255 = local read "Command Params"() -> (w399:string[][])
        n256 = Index Array(array=w403, index (row)=w400, index (col)=0) -> (element=w401:string)
        n257 = call <vilib>:"Invoke Commands.vi"("Command Params"=w399, "Function Name"=w401) -> ("Params"=w398:u8, "Started"=w393:bool)  [unwired: 7 in, 1 out]
        n258 = Array Subset(array=w399, length (row)=w398) -> (w397:string[][])  [unwired: 3 in]
        n259 = Select(t="Executing" ("Cmd Status"), s=w393, f="" ("Cmd Status")) -> (s? t:f=w394:string)
        n260 = local write "Cmd Status"(w394) -> ()
      }
      event "CheckList": Double Click {
        # "Shift clears all"
        # "Update symbols on the listbox"
        n261 = event-data() -> ("PlatMods.Shift"=w405:bool, "Row"=w407:i32)  [unwired: 1 in]
        n262 = case shown="True" w405 {
          tunnel: w407 -> [w411 _]
          tunnel: 1 -> [w410 _]
          frame False {
            n263 = property on="CheckList" class="LstBox (strict)"() -> ("Item Symbols"=w409:i32[])  [unwired: 2 in, 2 out]
            n264 = Replace Array Subset(array=w409, new element=w410, index=w411) -> (w408:i32[])
            n265 = property on="CheckList" class="LstBox (strict)"("Item Symbols"=w408) -> ()  [unwired: 2 in, 2 out]
          }
          frame True {
            w412 = 0 ("Top Row")
            n266 = property on="CheckList" class="LstBox (strict)"() -> ("Number of Rows"=w414:u32)  [unwired: 2 in, 2 out]
            n267 = Initialize Array(0, w414) -> (w413:i32[])
            n268 = property on="CheckList" class="LstBox (strict)"("Top Row"=w412, "Value"=w412, "Item Symbols"=w413) -> ()  [unwired: 2 in, 2 out]
          }
        }
      }
      event "CheckList": Key Down {
        # "Update symbols on the listbox\nLeft and right keys check and uncheck"
        n269 = event-data() -> ("VKey"=w418:T26)  [unwired: 1 in]
        n270 = case shown="\"Left\", \"Right\"" w418 {
          selector: w418 -> [w423 _]
          tunnel: eventvkey."Left" ("VKey") -> [w421 _]
          frame "Left", "Right" {
            n271 = Equal?(x=w421, y=w423) -> (x = y?=w422:bool)
            n272 = Select(t=0, s=w422, f=1) -> (s? t:f=w424:i32)
            n273 = property on="CheckList" class="LstBox (strict)"() -> ("Item Symbols"=w427:i32[])  [unwired: 2 in, 2 out]
            n274 = Replace Array Subset(array=w427, new element=w424, index="CheckList") -> (w426:i32[])
            n275 = property on="CheckList" class="LstBox (strict)"("Item Symbols"=w426) -> ()  [unwired: 2 in, 2 out]
          }
          frame Default {
          }
        }
      }
      event "Motor.Enable": Value Change {
        # "When the test mode otor enable helper is set, update that\ntree row item's value"
        n276 = event-data() -> ("NewVal"=w433:bool)  [unwired: 1 in]
        n277 = Unbundle("Motor") -> ("Value"=w432:dbl)  [unwired: 1 out]
        n278 = Select(t=w432, s=w433, f=0.0) -> (s? t:f=w430:dbl)
        n279 = call <vilib>:"NT Write Number.vi"("Numeric"=w430, "Name"=w429) -> ()  [unwired: 9 in, 1 out]
      }
      event "Test Slider": Value Change {
        # "When the test mode slider helper is set, update that\ntree row item's value"
        n280 = event-data() -> ("NewVal"=w436:dbl)  [unwired: 1 in]
        n281 = call <vilib>:"NT Write Number.vi"("Numeric"=w436, "Name"=w437) -> ()  [unwired: 9 in, 1 out]
      }
      event "On/Off": Value Change {
        # "When the test mode on/off helper value is set, update that\ntree row item's value"
        n282 = event-data() -> ("NewVal"=w441:bool)  [unwired: 1 in]
        n283 = Boolean To (0,1)(Boolean=w441) -> (0, 1=w440:i16)
        n284 = call <vilib>:"NT Write Number.vi"("Numeric"=w440, "Name"=w439) -> ()  [unwired: 9 in, 1 out]
      }
      event "Rev/Fwd": Value Change {
        # "When the test mode helper value for relays is set, update that\ntree row item's value"
        n285 = event-data() -> ("NewVal.Forward"=w449:bool, "NewVal.Reverse"=w448:bool)  [unwired: 1 in]
        n286 = Boolean To (0,1)(Boolean=w449) -> (0, 1=w445:i16)
        n287 = Boolean To (0,1)(Boolean=w448) -> (0, 1=w447:i16)
        n288 = Negate(x=w447) -> (-x=w446:i16)
        n289 = Add(x=w445, y=w446) -> (x+y=w444:i16)
        n290 = call <vilib>:"NT Write Number.vi"("Numeric"=w444, "Name"=w443) -> ()  [unwired: 9 in, 1 out]
      }
      event "Test Ring": Value Change {
        # "When a test mode helper value is selected from the ring,\nset the tree item's variable to the string value"
        n291 = event-data() -> ("NewVal"=w453:u16)  [unwired: 1 in]
        n292 = property on="Test Ring" class="Ring (strict)"() -> ("Strings []"=w454:string[])  [unwired: 2 in, 2 out]
        n293 = Index Array(array=w454, index=w453) -> (element=w452:string)
        n294 = call <vilib>:"NT Write String.vi"("String"=w452, "Name"=w451) -> ()  [unwired: 9 in, 1 out]
      }
      event "Rec Mode": Value Change {
        # "Update globals for recording mode and path to read log from.\nClear when logging and let NetworkTables set path for vision to\nuse."
        n295 = event-data() -> ("NewVal"=w465:enum32{"Stop", "Record", "Playback"})  [unwired: 1 in]
        n296 = global write "WPI_DashboardLogging Global.vi" "Logging Filename"(path "") -> ()
        n297 = global write "WPI_DashboardLogging Global.vi" "Recording"(w465) -> ()
        n298 = case shown="\"Playback\"" w465 {
          tunnel: w464 -> [_ w467 w476]
          tunnel: [_ _ w475] -> w462
          tunnel: [_ _ w474] -> _
          tunnel: w460 -> [_ _ w472]
          tunnel: cluster{i32, i32} {-250, 170} -> [_ _ w471]
          tunnel: [_ _ T27 {"Image Size"=TRUE, "Image Type"=TRUE, "Pixel Value"=TRUE, "ROI Information"=TRUE, "Zoom Factor"=FALSE} ("Image Information Shown:All Elements")] -> w455
          tunnel: [_ _ TRUE ("Zoom Factor")] -> w456
          tunnel: w458 -> [_ _ w468]
          frame Default {
          }
          frame "Stop", "Record" {
            # "Place Window too"
            n299 = invoke class="VI" method="FP.Close"(reference=w467) -> (reference out=w466:refnum<vi>)  [unwired: 2 in, 2 out]
            n300 = invoke class="VI" method="Abort VI"(reference=w466) -> ()  [unwired: 2 in, 3 out]
          }
          frame "Playback" {
            n301 = call "Open Playback Panel.vi"("Offset"=w471, "DB VI Ref"=w472, "Playback in"=w476) -> ("Playback out"=w473:refnum<vi>)  [unwired: 8 in]
            n302 = register-events(w473, w468) -> (reference out=w475:refnum<event-registration>, error out=w474:errorcluster)  [unwired: 2 in]
          }
        }
        n303 = property on="Camera Image Right" class="ImageControl"("Image Information Shown"=w455, "Image Information Visible"=w456) -> ()  [unwired: 2 in, 2 out]
        n304 = property on="Camera Image" class="ImageControl"("Image Information Shown"=w455, "Image Information Visible"=w456) -> ()  [unwired: 2 in, 2 out]
        n305 = call <vilib>:"WPI_DashboardNT Log FieldName Cache.vi"("Operation"=enum16{"Lookup/Add", "Index", "Clear"}."Clear") -> ()  [unwired: 8 in, 3 out]
      }
      event Panel Close {
        w478 = enum32{"Stop", "Record", "Playback"}."Stop" ("Rec Mode")
        # "Playback window has been closed, abort"
        n306 = event-data() -> ()  [unwired: 1 in, 4 out]
        n307 = local write "Rec Mode"(w478) -> ()
        n308 = global write "WPI_DashboardLogging Global.vi" "Recording"(w478) -> ()
      }
      event Panel Close {
        # "Abort playback window and ourself"
        n309 = event-data() -> ()  [unwired: 1 in, 4 out]
        n310 = invoke class="VI" method="FP.Close"(reference=w482) -> (reference out=w481:refnum<vi>)  [unwired: 2 in, 2 out]
        n311 = invoke class="VI" method="Abort VI"(reference=w481) -> (error out=w480:errorcluster)  [unwired: 2 in, 2 out]
        n312 = invoke class="VI" method="Abort VI"(error in=w480) -> ()  [unwired: 2 in, 3 out]
      }
      event User Event {
        n313 = event-data() -> ("IDs"=w489:cluster{"RPC field ID":u16, "Unique ID":u16}, "String"=w488:string)  [unwired: 1 in]
        n314 = Bundle("IDs"=w489, "String"=w488) -> (w487:T13)  [unwired: 1 in]
        n315 = call <vilib>:"Retrieve RPC Response.vi"("RPC Response"=w487) -> ("Output"=w485:string[][])  [unwired: 10 in]
        n316 = Build Array (concatenate)(w483, w485) -> (w484:string[][])
        n317 = local write "Command Params"(w484) -> ()
        n318 = local write "Cmd Status"("" ("Cmd Status")) -> ()
      }
      event "Tree": Double Click {
        n319 = event-data() -> ("PlatMods"=w495:T30, "Tag"=w492:string)  [unwired: 1 in]
        n320 = Unbundle(w495) -> ("Shift"=w494:bool)  [unwired: 4 out]
        n321 = String Subset(string=w492, length (rest)=1 ("length (rest)")) -> (substring=w491:string)  [unwired: 1 in]
        n322 = Not(x=w494) -> (.not. x?=w493:bool)
        n323 = case shown="\"/\"" w491 {
          tunnel: w492 -> [_ w498]
          tunnel: w493 -> [_ w497]
          frame Default {
          }
          frame "/" {
            n324 = call <vilib>:"NT Update Persistence.vi"("Persistence"=w497, "Name"=w498) -> ()  [unwired: 9 in, 1 out]
          }
        }
      }
    }
  }
  n325 = while {
    tunnel: w64 -> [w500]
    i -> [w503]
    stop <- FALSE stop-if-true
    n326 = Wait (ms)(milliseconds to wait=u32 100) -> ()  [unwired: 1 out]
    n327 = case shown="\"Playback\"" "Rec Mode" {
      tunnel: w503 -> [_ _ w518]
      tunnel: [u32 2829099 ("Base Color") u32 11141120 ("Target Color") w507] -> w499
      frame "Stop", Default {
        # "Reset the color, extra updates don't cost much"
      }
      frame "Record" {
      }
      frame "Playback" {
        # "Playback"
        n328 = Quotient & Remainder(x=w518, y=u32 50 ("milliseconds to wait")) -> (x-y*floor(x/y)=w514:u32)  [unwired: 1 out]
        n329 = Divide(x=w514, y=u32 50 ("milliseconds to wait")) -> (x/y=w511:dbl)
        n330 = Multiply(x=6.283185307179586, y=w511) -> (x*y=w516:dbl)
        n331 = Sine(x=w516) -> (sin(x)=w515:dbl)
        n332 = Absolute Value(x=w515) -> (abs(x)=w508:dbl)
        n333 = call "Interpolate RGB Color.vi"("Proportion"=w508, "Target Color"=u32 30976, "Base Color"=u32 2829099) -> ("Result Color"=w507:u32)  [unwired: 8 in]
      }
    }
    n334 = property class="Pane"(reference=w500, "PaneColor"=w499) -> ()  [unwired: 1 in, 2 out]
  }
  n335 = property on="On/Off" class="Bool (strict)"("Visible"=w35) -> ()  [unwired: 2 in, 2 out]
  n336 = property on="Motor" class="Clust (strict)"("Visible"=w35) -> ()  [unwired: 2 in, 2 out]
  n337 = property on="Progress" class="Clust (strict)"("Visible"=w35) -> ()  [unwired: 2 in, 2 out]
  n338 = property on="Test Ring" class="Ring (strict)"("Visible"=w35) -> ()  [unwired: 2 in, 2 out]
  n339 = property on="Rev/Fwd" class="Clust (strict)"("Visible"=w35) -> ()  [unwired: 2 in, 2 out]
  n340 = while {
    tunnel: u16 1741 ("timeout ms (25000)") -> [w520]
    stop <- FALSE stop-if-true
    n341 = TCP Create Listener(10:w520) -> (0:w519:errorcluster, 3:w521:refnum<k5>)  [unwired: 4 in, 1 out]
    n342 = case shown="No Error" w519 {
      selector: w519 -> [w523 _]
      tunnel: w521 -> [w524 _]
      frame No Error {
        n343 = while {
          tunnel: w524 -> [w527]
          tunnel: w523 -> [w526]
          stop <- FALSE stop-if-true
          n344 = TCP Wait On Listener(8:w526, 11:w527) -> (0:w528:errorcluster, 4:w529:refnum<k5>)  [unwired: 2 in, 3 out]
          n345 = local write "TCP"(w529) -> ()
          n346 = case shown="No Error" w528 {
            frame No Error {
            }
            frame Error {
              n347 = Wait (ms)(milliseconds to wait=u32 1000) -> ()  [unwired: 1 out]
            }
          }
        }
      }
      frame Error {
        n348 = Wait (ms)(milliseconds to wait=u32 1000) -> ()  [unwired: 1 out]
      }
    }
  }
  n349 = local write "Command Selection"(u16 0 ("milliseconds to wait")) -> ()
  n350 = local write "Command Params"(string[][] [] ("Command Params")) -> ()
  n351 = global write "WPI_DashboardLogging Global.vi" "Recording"(w58) -> ()
  n352 = local write "Rec Mode"(w58) -> ()
  n353 = call <vilib>:"NT Write String.vi"("String"="Select Auto", "Name"="Auto Selector") -> ()  [unwired: 9 in, 1 out]
